vi "prepXYscan.vi"   [LabVIEW 2013]
uses:
  <vilib>/DAQmx/write.llb/DAQmx Write (Analog 2D DBL NChan NSamp).vi
  <vilib>/DAQmx/create/channels.llb/DAQmx Create Channel (AO-Voltage-Basic).vi
  <vilib>/DAQmx/configure/timing.llb/DAQmx Timing (Sample Clock).vi
  <vilib>/DAQmx/miscellaneous.llb/DAQmx Fill In Error Info.vi
types:
  T1 = cluster{"CH1 AI":tag, "CH1 CI":tag, "CH2 AI":tag, "CH2 CI":tag, "AI X":tag, "AI Y":tag, "AO X-Y":tag, "CH1ST":bool, "CH2ST":bool, "Sigcase":i16, "StageS":i32, "StageL":i32, "data dir":path, "AI VC":tag, "AI CC":tag, "AO CWlaser":tag, "AO VtoP":tag, "shutter":tag, "488":tag, "532":tag, "640":tag}
  T2 = cluster{"Xpixels":i32, "Vx-min ref":dbl, "Vx-max ref":dbl, "Ypixels":i32, "Vy-min ref":dbl, "Vy-max ref":dbl, "srate":dbl, "type":string, "date":string, "time":string, "Colormap":u16, "square pixels":bool, "square matrix":bool, "Xpixels Img":i32, "Vx-min Img":dbl, "VX-max Img":dbl, "Ypixels Img":i32, "Vy-min Img":dbl, "Vy-max Img ":dbl, "autoshutter":bool, "P":dbl, "sAOxy":i32, "finite":bool, "cont":bool, "wavdet":bool, "measpoints":i32, "avpp":i32, "bufferAO":i32, "bufferAI":i32, "CH1":bool, "CH2":bool, "X":bool, "Y":bool, "timeout":dbl, "starttick":u32, "waveform":path, "Vy-ref":dbl, "Vx-ref":dbl, "refreshrate":dbl, "refreshbuffer":i32, "tt_cycles":i32, "motorref":refnum<k7>, "mirrorswitch":refnum<k7>, "sample mode":i32}
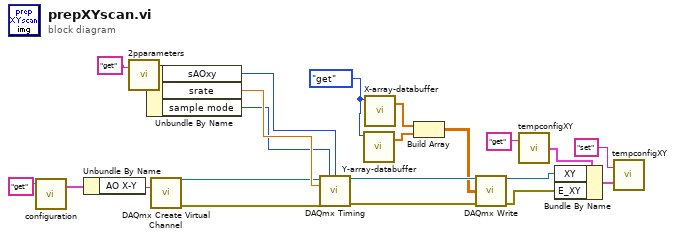
[diagram p0: block diagram]
diagram:
  w8 = enum16{"get", "set", "clear", "append"}."get" ("command")
  n1 = call "configuration.vi"("command"="get") -> ("config out"=w10:T1)  [unwired: 2 in, 1 out]
  n2 = Unbundle By Name(w10) -> ("AO X-Y"=w12:tag)
  n3 = call "2pparameters.vi"("command"="get") -> ("Params out"=w14:T2)  [unwired: 1 in]
  n4 = Unbundle By Name(w14) -> ("sAOxy"=w15:i32, "srate"=w22:dbl, "sample mode"=w1:i32)
  n5 = call-poly <vilib>:"DAQmx Create Virtual Channel.vi"("physical channels"=w12) -> ("task out"=w6:refnum<k21>, "error out"=w5:errorcluster)  [unwired: 13 in]
  n6 = call-poly <vilib>:"DAQmx Timing.vi"("task/channels in"=w6, "sample mode"=w1, "samples per channel"=w15, "rate"=w22, "error in"=w5) -> ("task out"=w4:refnum<k21>, "error out"=w2:errorcluster)  [unwired: 9 in]
  n7 = call "Y-array-databuffer.vi"("command"=w8) -> ("array out"=w9:dbl[])  [unwired: 3 in, 1 out]
  n8 = call "X-array-databuffer.vi"("command"=w8) -> ("array out"=w7:dbl[])  [unwired: 3 in, 1 out]
  n9 = Build Array(w7, w9) -> (w3:dbl[][])
  n10 = call-poly <vilib>:"DAQmx Write.vi"("task/channels in"=w4, "data"=w3, "error in"=w2) -> ("task out"=w17:refnum<k21>, "error out"=w16:errorcluster)  [unwired: 10 in, 1 out]
  n11 = call "tempconfigXY.vi"("command"="get") -> ("Temp Config out"=w19:cluster{" XY":refnum<k21>, "E_XY":errorcluster})  [unwired: 1 in]
  n12 = Bundle By Name(cluster=w19, "XY"=w17, "E_XY"=w16) -> (w20:cluster{" XY":refnum<k21>, "E_XY":errorcluster})
  n13 = call "tempconfigXY.vi"("Temp Config in"=w20, "command"="set") -> ()  [unwired: 1 out]
